vi "上下限.vi"(1 "要比较的":dbl, 2 "范围的中心":dbl) -> (0 "T/F":bool)   [LabVIEW 2013]
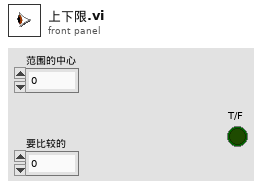
[diagram p1: front panel]
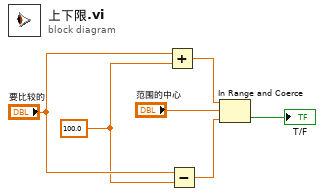
[diagram p0: block diagram]
diagram:
  w1 = 100.0 ("范围的中心 2")
  n1 = Add(x="要比较的", y=w1) -> (x+y=w5:dbl)
  n2 = Subtract(x="要比较的", y=w1) -> (x-y=w4:dbl)
  n3 = In Range and Coerce(upper limit=w5, x="范围的中心", lower limit=w4) -> (In Range?=→"T/F":bool)  [unwired: 1 out]
